vi "EventKick.vi"(0 "Toque":bool, 1 "id":dbl, 2 "IA State Input":T1) -> (8 "Kick":bool)   [LabVIEW 2017]
uses:
  Core/AI Input.ctl
  Core/AI Robot.ctl
  Intel/Functions Enum.ctl
  Intel/AttackerStates.ctl
  Core/AI Ball.ctl
  Core/Field Size.ctl
  Core/AI Judge.ctl
  Intel/Command Enum.ctl
  Events.ctl
panel:
  out "Boolean":bool
  in  "Dist":dbl=200.0
  in  "Time":u32=200
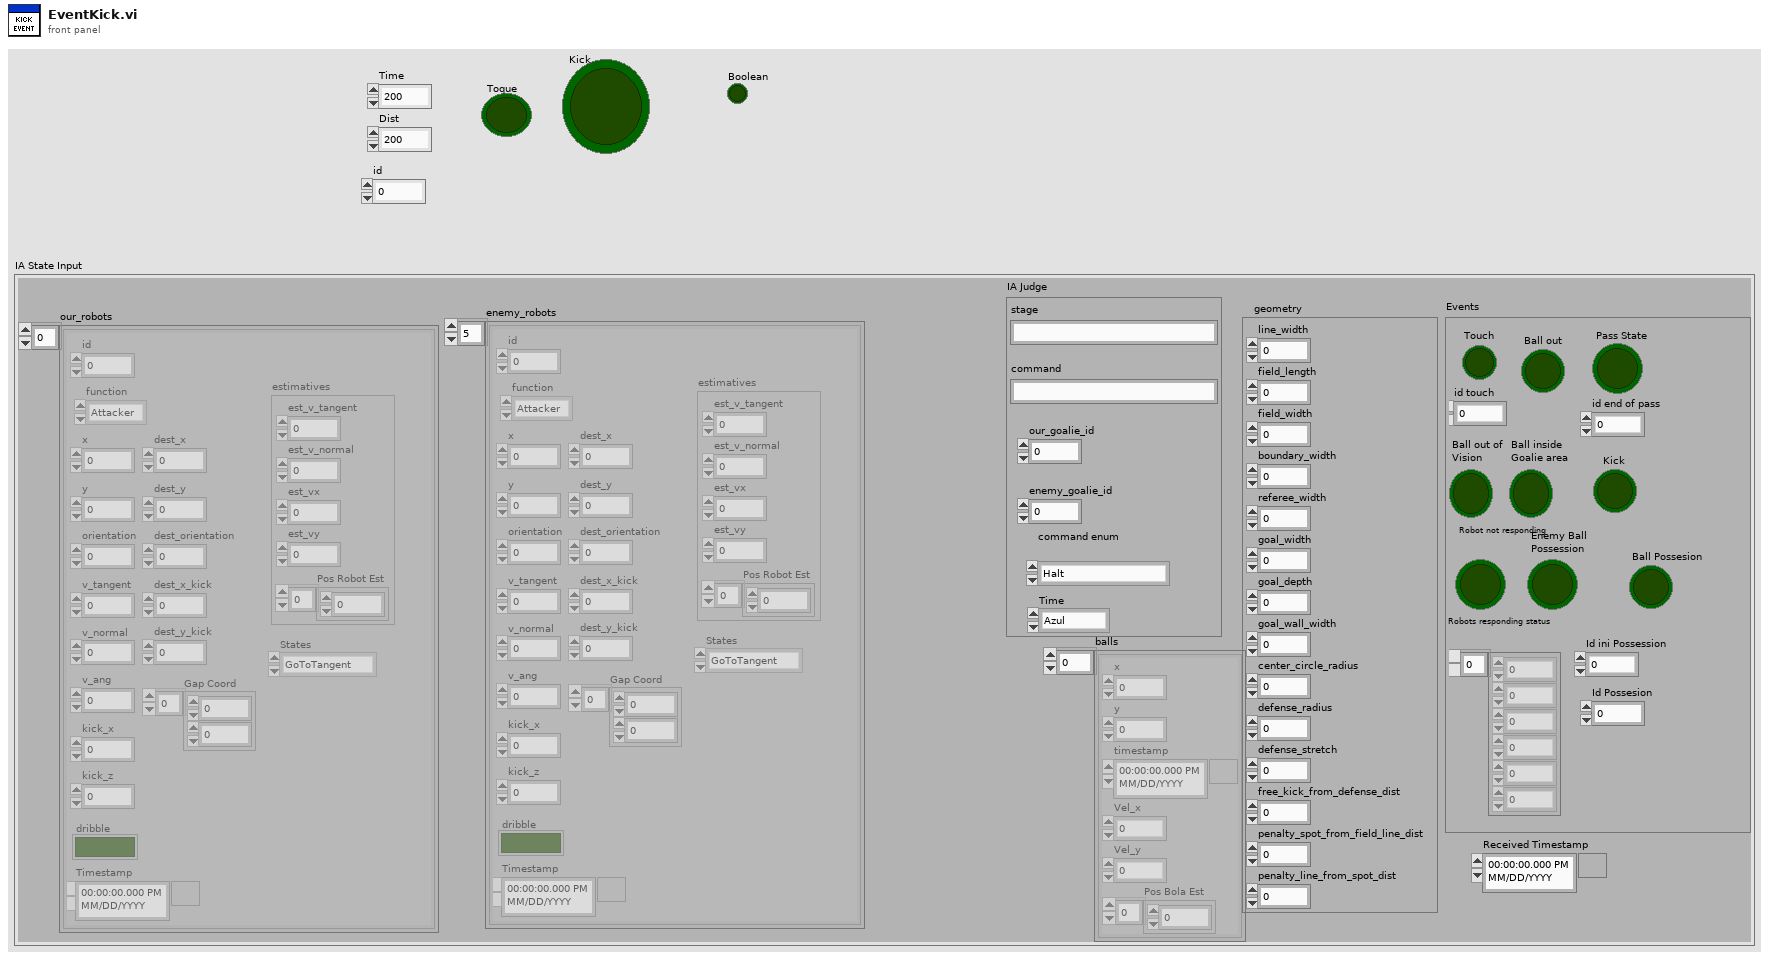
[diagram p1: front panel]
types:
  T1 = typedef "AI Input.ctl" = cluster{"our_robots":T2[], "enemy_robots":T2[], "balls":T5[], "geometry":T6, "IA Judge":T7, "Received Timestamp":timestamp, "Events":T9}
  T2 = typedef "AI Robot.ctl" = cluster{"id":u32, "function":T3, "x":dbl, "y":dbl, "orientation":dbl, "v_tangent":dbl, "v_normal":dbl, "v_ang":dbl, "kick_x":dbl, "kick_z":dbl, "dribble":bool, "Timestamp":timestamp, "dest_x":dbl, "dest_y":dbl, "dest_orientation":dbl, "estimatives":cluster{"est_v_tangent":dbl, "est_v_normal":dbl, "est_vx":dbl, "est_vy":dbl, "Pos Robot Est":dbl[]}, "dest_x_kick":dbl, "dest_y_kick":dbl, "Gap Coord":dbl[], "States":T4}
  T3 = typedef "Functions Enum.ctl" = enum16{"Attacker", "Goalie", "Defender", "Striker", "Goto 0", "Dummy", "Kicker", "ZigZag"}
  T4 = typedef "AttackerStates.ctl" = enum16{"Pass", "GoToTangent", "BallGetting", "GoToKick", ""}
  T5 = typedef "AI Ball.ctl" = cluster{"x":dbl, "y":dbl, "timestamp":timestamp, "Vel_x":dbl, "Vel_y":dbl, "Pos Bola Est":dbl[]}
  T6 = typedef "Field Size.ctl" = cluster{"line_width":u32, "field_length":u32, "field_width":u32, "boundary_width":u32, "referee_width":u32, "goal_width":u32, "goal_depth":u32, "goal_wall_width":u32, "center_circle_radius":u32, "defense_radius":u32, "defense_stretch":u32, "free_kick_from_defense_dist":u32, "penalty_spot_from_field_line_dist":u32, "penalty_line_from_spot_dist":u32}
  T7 = typedef "AI Judge.ctl" = cluster{"stage":string, "command":string, "our_goalie_id":dbl, "enemy_goalie_id":dbl, "command enum":T8, "Time":enum16{"Azul", "Amarelo"}}
  T8 = typedef "Command Enum.ctl" = enum16{"Halt", "Stop", "Force Start", "PKA Normal Start", "Prepare Kickoff Ally", "PKE Normal Start", "Prepare Kickoff Enemy", "Prepare Penalty Ally", "PPA Normal Start", "Prepare Penalty Enemy", "PPE Normal Start", "Direct Free Enemy", "Direct Free Ally", "Indirect Free Enemy", "Indirect Free Ally", "Timeout Enemy", "Timeout Ally", "Goal Enemy", "Goal Ally", "Ball Placement Enemy", "Ball Placement Ally", "Normal Half Time", "Extra Time Break", "Extra Half Time", "None", "Post Game"}
  T9 = typedef "Events.ctl" = cluster{"Touch":bool, "Ball out":bool, "id touch":dbl, "Ball out of \nVision":bool, "Ball inside \nGoalie area":bool, "Robot not responding":bool, "Robots responding status":dbl[], "Enemy Ball \nPossession":bool, "Pass State":bool, "id end of pass":dbl, "Kick":bool, "Id ini Possession":dbl, "Ball Possesion":bool, "Id Possesion":dbl}
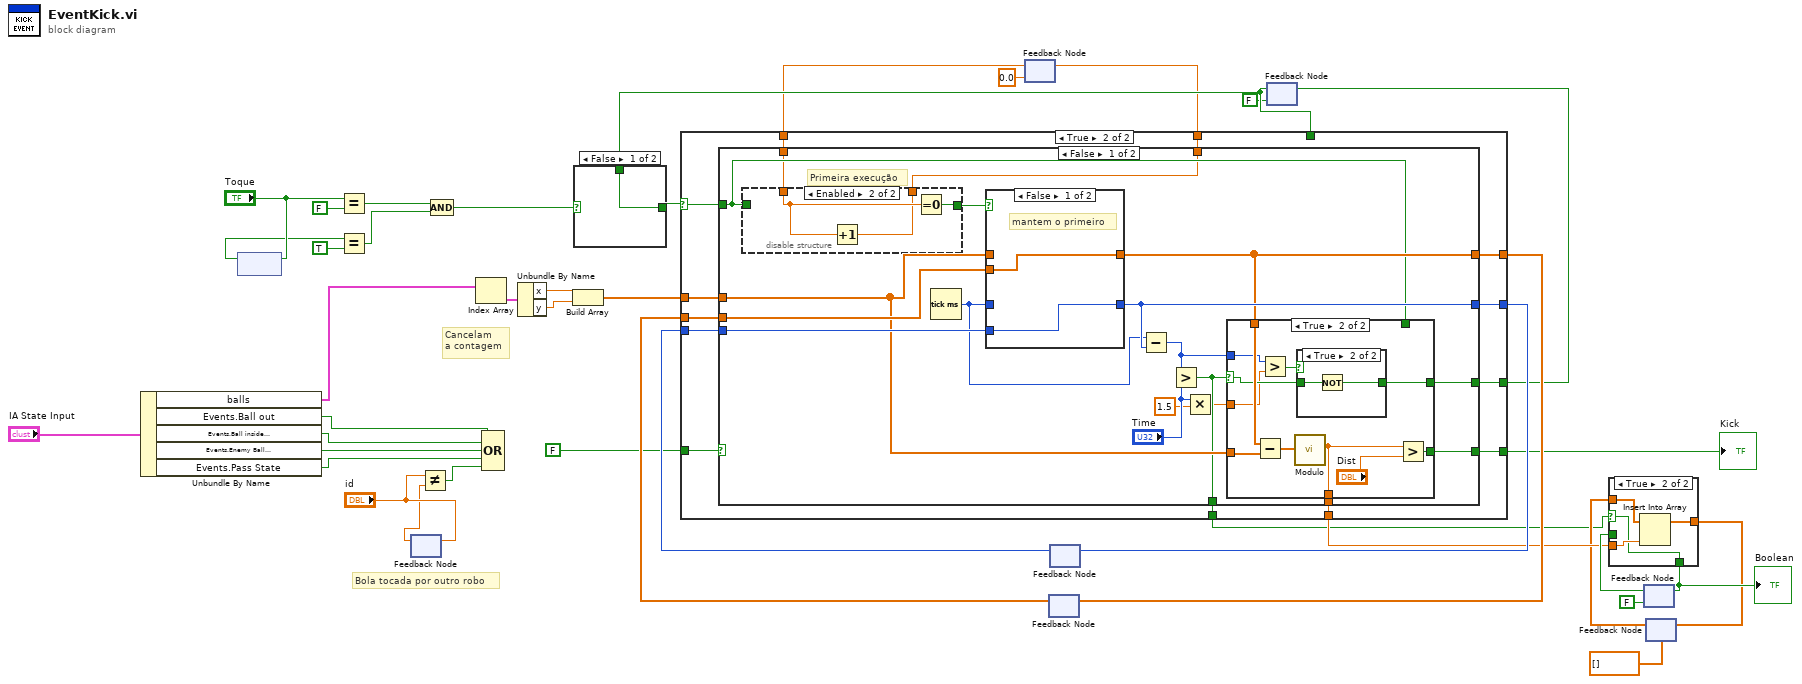
[diagram p0: block diagram]
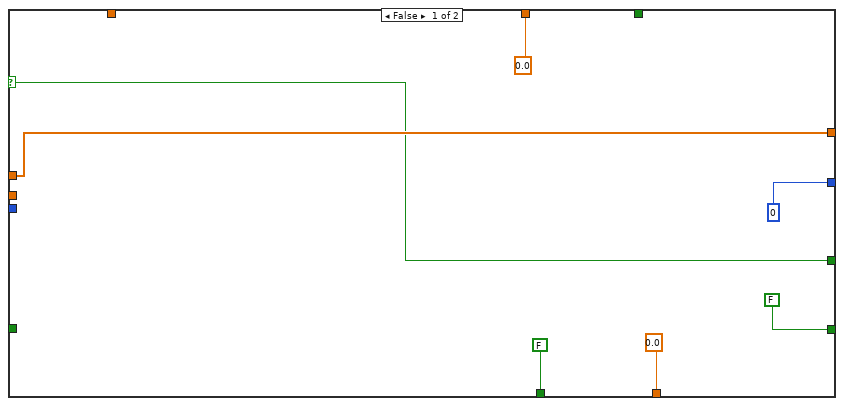
[diagram p4: hidden frame]
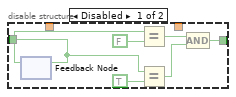
[diagram p5: hidden frame]
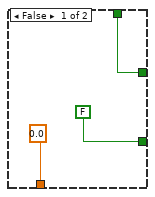
[diagram p6: hidden frame]
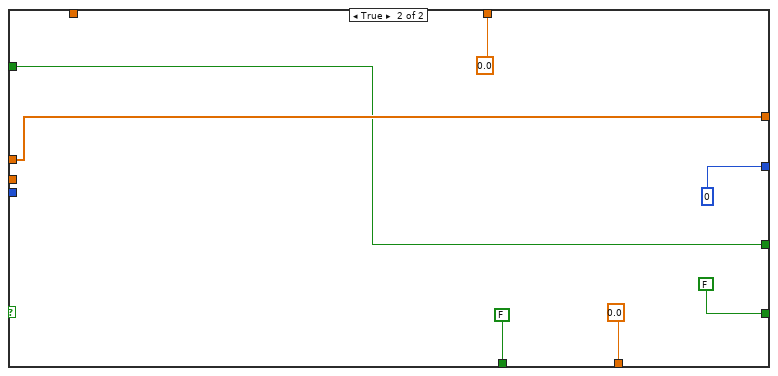
[diagram p9: hidden frame]
diagram:
  # "Cancelam \na contagem"
  # "Bola tocada por outro robo"
  n1 = Unbundle By Name("IA State Input") -> ("balls"=w27:T5[], "Events.Ball out"=w34:bool, "Events.Ball inside \nGoalie area"=w33:bool, "Events.Enemy Ball \nPossession"=w32:bool, "Events.Pass State"=w31:bool)
  n2 = feedback #1() -> (w37:bool)  [unwired: 1 in]
  n3 = feedback-in #1("Toque") -> ()
  n4 = Equal?(x="Toque", y=FALSE) -> (x = y?=w40:bool)
  n5 = Equal?(x=w37, y=TRUE) -> (x = y?=w39:bool)
  n6 = feedback #2() -> (w29:dbl)  [unwired: 1 in]
  n7 = feedback-in #2("id") -> ()
  n8 = Not Equal?(x="id", y=w29) -> (x != y?=w28:bool)
  n9 = Compound Arithmetic op=AND(w40, w39) -> (w16:bool)
  n10 = Index Array(array=w27) -> (element=w26:T5)  [unwired: 1 in]
  n11 = Compound Arithmetic op=OR(w34, w33, w32, w31, w28) -> ()  [unwired: 1 out]
  n12 = Unbundle By Name(w26) -> ("x"=w25:dbl, "y"=w24:dbl)
  n13 = Build Array(w25, w24) -> (w23:dbl[])
  n14 = feedback #3(0.0 ("Numeric")) -> (w3:dbl)
  n15 = feedback #4() -> (w21:dbl[])  [unwired: 1 in]
  n16 = feedback #5() -> (w19:u32)  [unwired: 1 in]
  n17 = feedback #6(FALSE) -> (w17:bool)
  n18 = case shown="False" w16 {
    selector: w16 -> [_ w43]
    tunnel: w17 -> [w42 _]
    tunnel: [w42 w43] -> w15
    frame False {
    }
    frame True {
    }
  }
  n19 = case shown="True" w15 {
    selector: w15 -> [w47 w63]
    tunnel: w23 -> [w50 w59]
    tunnel: [w50 w58] -> w22
    tunnel: w21 -> [_ w62]
    tunnel: [u32 0 ("millisecond timer value") w60] -> w20
    tunnel: w19 -> [_ w61]
    tunnel: [FALSE w57] -> w13
    tunnel: FALSE -> [_ w56]
    tunnel: [w47 w55] -> w18
    tunnel: w17 -> [_ _]
    tunnel: [0.0 ("Modulo") w54] -> w8
    tunnel: [FALSE w53] -> w4
    tunnel: w3 -> [_ w52]
    tunnel: [0.0 w51] -> w1
    frame False {
    }
    frame True {
      n20 = case shown="False" w56 {
        tunnel: w63 -> [w72 w116]
        tunnel: w62 -> [w80 _]
        tunnel: w61 -> [w79 _]
        tunnel: [w78 u32 0 ("millisecond timer value")] -> w60
        tunnel: w59 -> [w76 w119]
        tunnel: [w75 w119] -> w58
        tunnel: [w74 FALSE] -> w57
        tunnel: [w73 w116] -> w55
        tunnel: [w71 0.0 ("Modulo")] -> w54
        tunnel: [w70 FALSE] -> w53
        tunnel: w52 -> [w69 _]
        tunnel: [w68 0.0] -> w51
        frame False {
          # "Primeira execução"
          n21 = disable-structure shown="Enabled" {
            disable-tunnel: [w83 w91] -> w81
            disable-tunnel: w72 -> [w82 _]
            disable-tunnel: w69 -> [_ w90]
            disable-tunnel: [_ w89] -> w68
            frame Disabled {
              n22 = feedback #7() -> (w84:bool)  [unwired: 1 in]
              n23 = feedback-in #7(w82) -> ()
              n24 = Equal?(x=w84, y=FALSE) -> (x = y?=w88:bool)
              n25 = Equal?(x=w82, y=TRUE) -> (x = y?=w87:bool)
              n26 = Compound Arithmetic op=AND(w88, w87) -> (w83:bool)
            }
            frame Enabled {
              n27 = Increment(x=w90) -> (x+1=w89:dbl)
              n28 = Equal To 0?(x=w90) -> (x = 0?=w91:bool)
            }
          }
          n29 = Tick Count (ms)() -> (millisecond timer value=w77:u32)
          n30 = case shown="False" w81 {
            tunnel: w76 -> [_ w112]
            tunnel: [w110 w112] -> w75
            tunnel: w80 -> [w110 _]
            tunnel: [w109 w111] -> w78
            tunnel: w77 -> [_ w111]
            tunnel: w79 -> [w109 _]
            frame False {
              # "mantem o primeiro"
            }
            frame True {
              # "atualiza o valor do \nprimeiro"
            }
          }
          n31 = Subtract(x=w77, y=w78) -> (x-y=w67:u32)
          n32 = Greater?(x=w67, y="Time") -> (0:w70:bool)
          n33 = Multiply(x="Time", y=1.5) -> (x*y=w64:dbl)
          n34 = case shown="True" w70 {
            selector: w70 -> [_ w100]
            tunnel: w76 -> [_ w105]
            tunnel: w75 -> [_ w104]
            tunnel: [FALSE w101] -> w74
            tunnel: [w93 w99] -> w73
            tunnel: w72 -> [w93 _]
            tunnel: [0.0 ("Modulo") w98] -> w71
            tunnel: w67 -> [_ w97]
            tunnel: w64 -> [_ w96]
            frame False {
            }
            frame True {
              n35 = Subtract(x=w104, y=w105) -> (x-y=w103:dbl[])
              n36 = Greater?(x=w97, y=w96) -> (0:w95:bool)
              n37 = call "Modulo.vi"("2D vector"=w103) -> ("Modulo"=w98:dbl)  [unwired: 10 in]
              n38 = case shown="True" w95 {
                tunnel: w100 -> [w106 w108]
                tunnel: [w106 w107] -> w99
                frame False {
                }
                frame True {
                  n39 = Not(x=w108) -> (.not. x?=w107:bool)
                }
              }
              n40 = Greater?(x=w98, y="Dist") -> (0:w101:bool)
            }
          }
        }
        frame True {
        }
      }
    }
  }
  "Kick" <- w13
  n41 = feedback-in #3(w1) -> ()
  n42 = feedback-in #4(w22) -> ()
  n43 = feedback-in #5(w20) -> ()
  n44 = feedback-in #6(w18) -> ()
  n45 = feedback #8(FALSE) -> (w11:bool)
  n46 = feedback #9(dbl[] []) -> (w6:dbl[])
  n47 = case shown="True" w4 {
    selector: w4 -> [_ w122]
    tunnel: [w120 w122] -> w12
    tunnel: w11 -> [w120 _]
    tunnel: w8 -> [_ w125]
    tunnel: [w121 w124] -> w7
    tunnel: w6 -> [w121 w123]
    frame False {
    }
    frame True {
      n48 = Insert Into Array(array=w123, new element=w125) -> (w124:dbl[])  [unwired: 1 in]
    }
  }
  "Boolean" <- w12
  n49 = feedback-in #8(w12) -> ()
  n50 = feedback-in #9(w7) -> ()
